vi "Server Data FGV.vi"(7 "mode":enum16{"get", "set", "reset"}(ring), 8 "error in":errorcluster, 10 "data in":variant, 11 "name (empty=auto)":string) -> (0 "error out":errorcluster, 1 "exists?":bool, 2 "data out":variant, 3 "name out":string)   [LabVIEW 2026, in "G-AI Core.lvlib"]
doc: "Stores the variant lookup table with VI references or other references that need to be stored perpetually."
uses:
  G-AI Core.lvlib
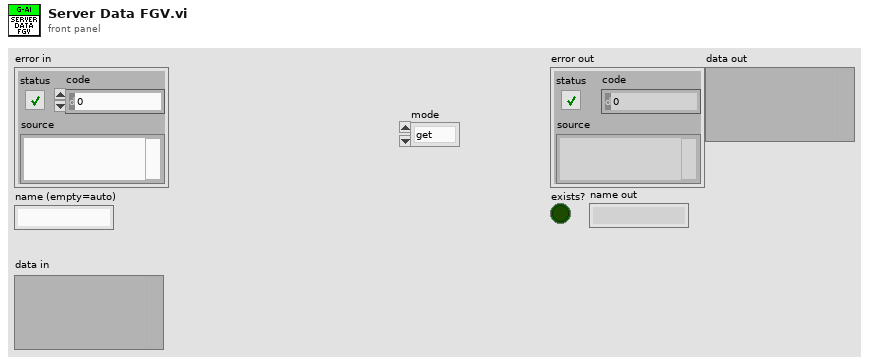
[diagram p1: front panel]
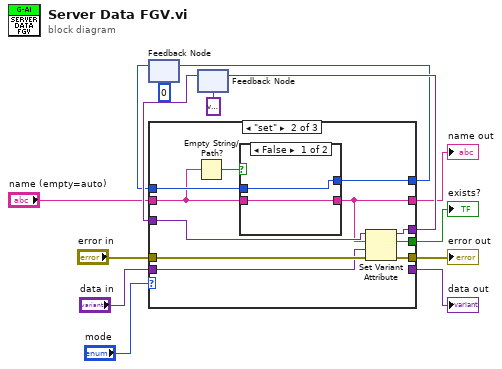
[diagram p0: block diagram]
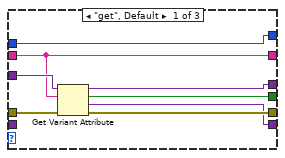
[diagram p2: hidden frame]
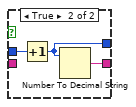
[diagram p3: hidden frame]
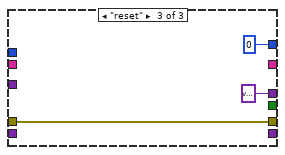
[diagram p4: hidden frame]
diagram:
  n1 = feedback #1(0) -> (w4:i32)
  n2 = feedback #2(variant ("Variant out")) -> (w12:variant)
  n3 = case shown="\"set\"" "mode" {
    tunnel: [w19 w32 variant] -> w13
    tunnel: w12 -> [w20 w33 _]
    tunnel: [w21 w31 w40] -> w11
    tunnel: "error in" -> [w22 w30 w40]
    tunnel: "name (empty=auto)" -> [w15 w24 _]
    tunnel: "data in" -> [_ w29 _]
    tunnel: [w18 w28 _] -> w7
    tunnel: [w17 _ _] -> w6
    tunnel: [w16 w26 0] -> w5
    tunnel: w4 -> [w16 w27 _]
    tunnel: [w15 w23 _] -> w3
    frame "get", Default {
      n4 = Get Variant Attribute(Variant=w20, name=w15, error in=w22) -> (duplicate Variant=w19:variant, found=w18:bool, value=w17:variant, error out=w21:errorcluster)  [unwired: 1 in]
    }
    frame "set" {
      n5 = Empty String/Path?(string/path=w24) -> (empty?=w25:bool)
      n6 = case shown="False" w25 {
        tunnel: w27 -> [w35 w38]
        tunnel: [w35 w37] -> w26
        tunnel: [w34 w36] -> w23
        tunnel: w24 -> [w34 _]
        frame False {
        }
        frame True {
          n7 = Increment(x=w38) -> (x+1=w37:i32)
          n8 = Number To Decimal String(number=w37) -> (decimal integer string=w36:string)  [unwired: 1 in]
        }
      }
      n9 = Set Variant Attribute(Variant=w33, name=w23, value=w29, error in=w30) -> (Variant out=w32:variant, replaced=w28:bool, error out=w31:errorcluster)
    }
    frame "reset" {
    }
  }
  "error out" <- w11
  "exists?" <- w7
  "data out" <- w6
  "name out" <- w3
  n10 = feedback-in #1(w5) -> ()
  n11 = feedback-in #2(w13) -> ()
